vi "ELTA_Ethernet_CMD.vi"(5 "ELTA_Ethernet_Func":T2, 7 "timeout ms":i32=25000, 8 "error in":errorcluster, 11 "CMD in":string) -> (0 "error out":errorcluster, 2 "Response? (00)":bool, 3 "data out":string)   [LabVIEW 2023, in "ELTA.lvlib"]
uses:
  ELTA.lvlib
  DUT_ctrl.ctl
panel:
  in  "TCPIPin":T1={"address"="192.168.100.111", "remote port or service name"=5025, "timeout ms "=10000}
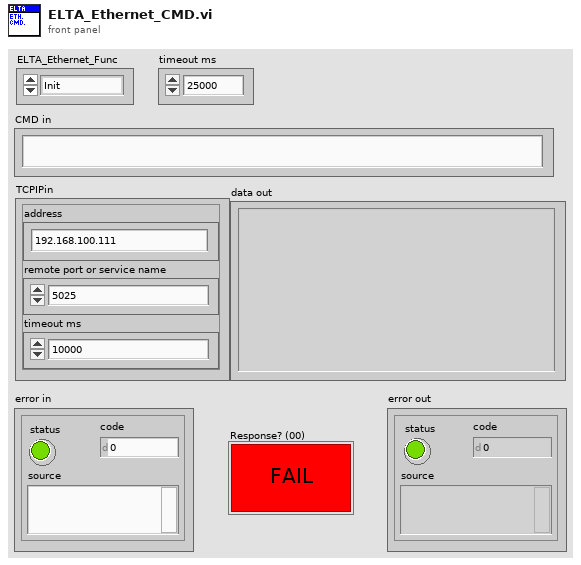
[diagram p1: front panel]
types:
  T1 = cluster{"address":string, "remote port or service name":u16, "timeout ms ":i32}
  T2 = typedef "ELTA.lvlib/DUT_ctrl.ctl" = enum16{"Init", "Close", "CMD"}
  T3 = enum16{"Standard", "Buffered", "CRLF", "Immediate"}
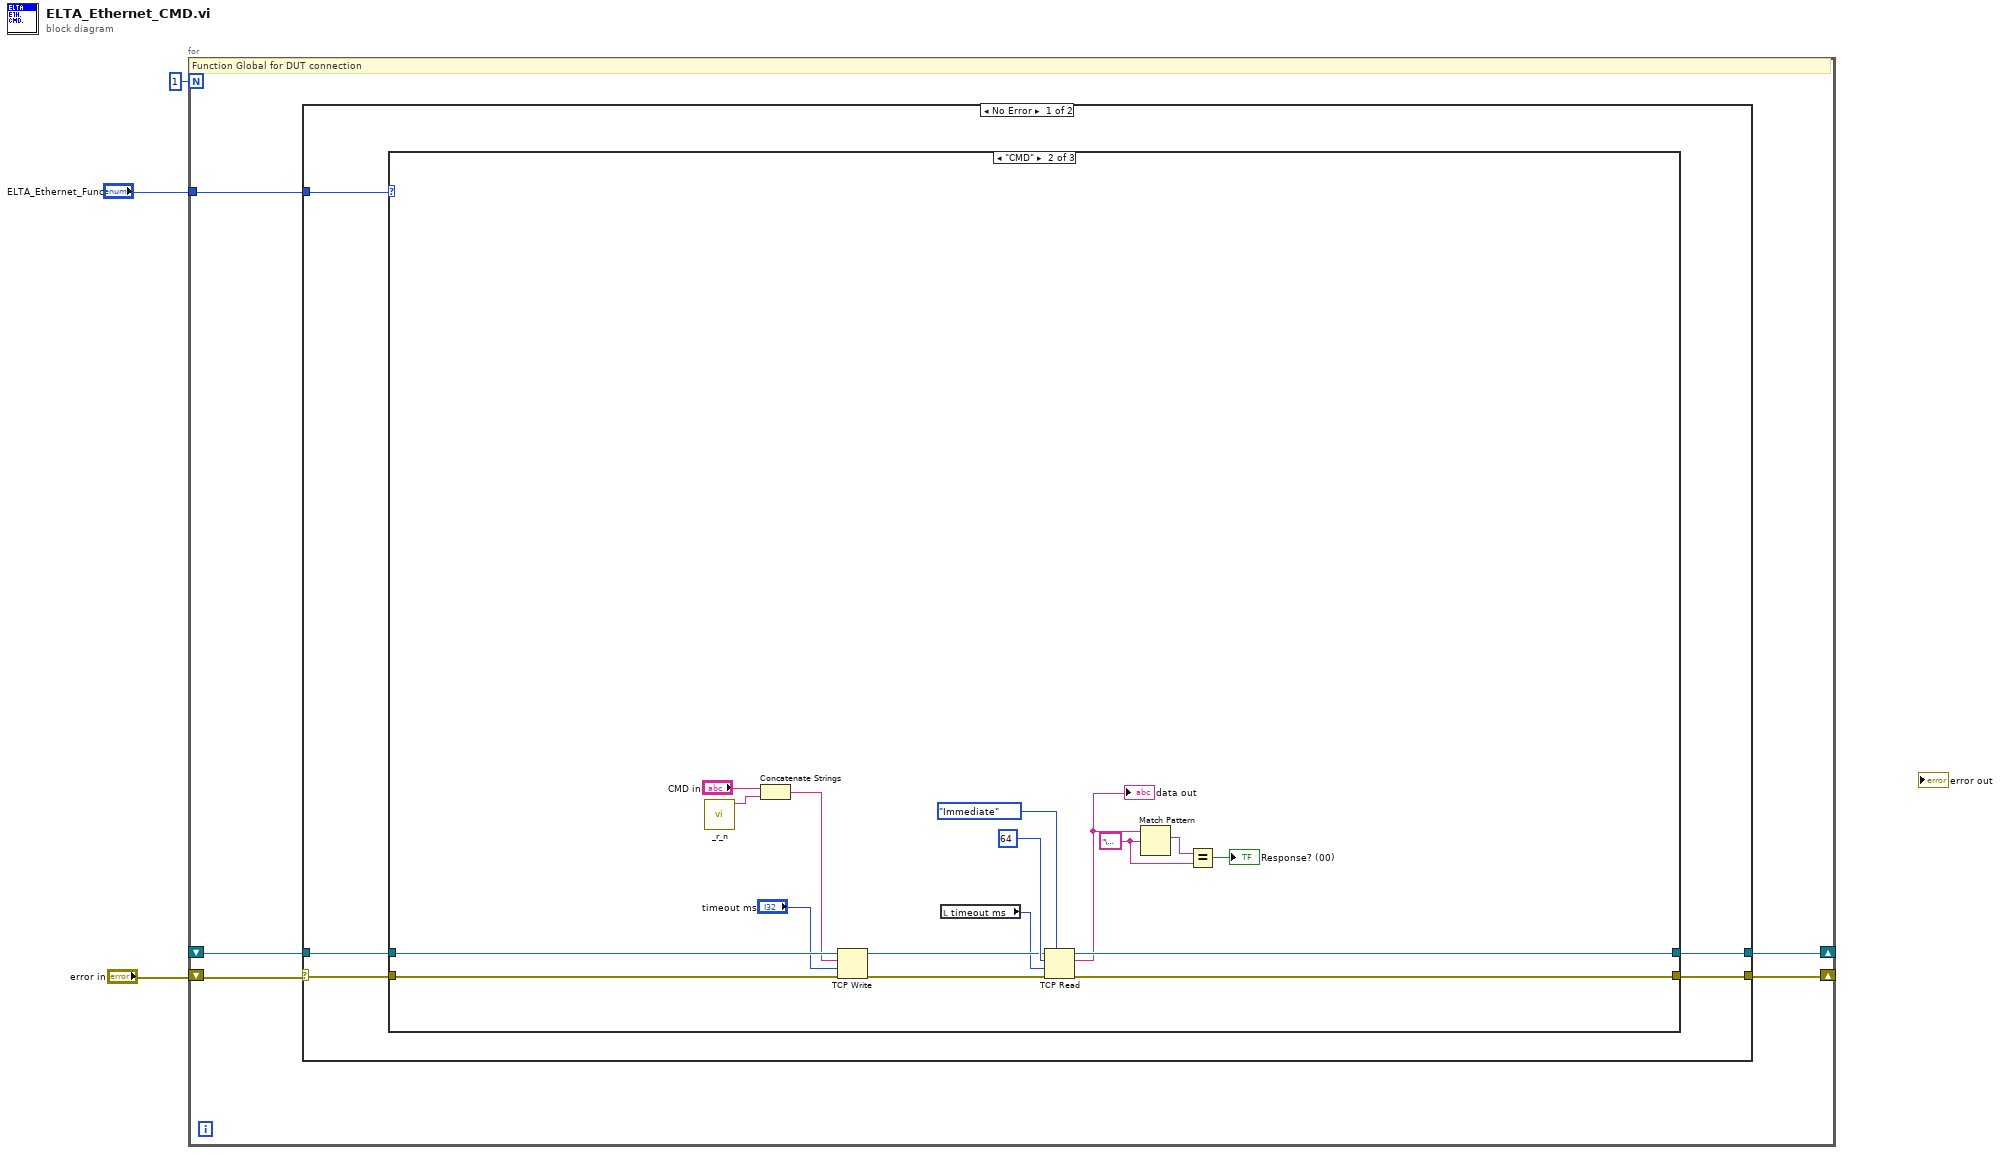
[diagram p0: block diagram]
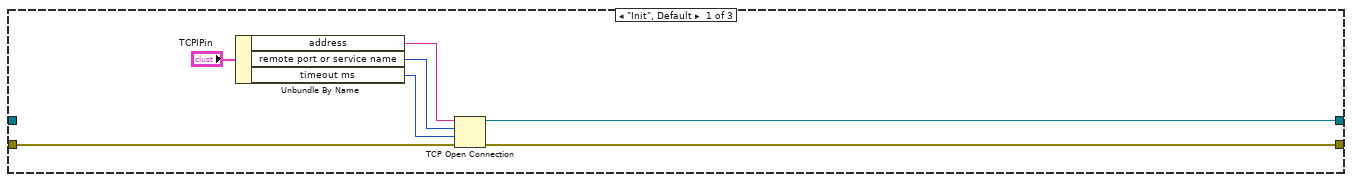
[diagram p2: hidden frame]
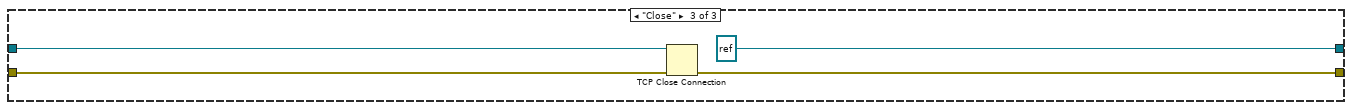
[diagram p3: hidden frame]
diagram:
  n1 = for {
    N: 1 -> [_]
    tunnel: "ELTA_Ethernet_Func" -> [w7]
    shift-right: [w6] -> _
    shift-left: "error in" -> [w8]
    shift-right: [w5] -> _
    shift-left: _ -> [w4]
    # "Function Global for DUT connection"
    n2 = case shown="No Error" w8 {
      selector: w8 -> [w13 w43]
      tunnel: w7 -> [w12 _]
      tunnel: [w11 w43] -> w6
      tunnel: [w10 w42] -> w5
      tunnel: w4 -> [w9 w42]
      frame No Error {
        n3 = case shown="\"CMD\"" w12 {
          tunnel: w13 -> [w19 w37 w40]
          tunnel: [w15 w28 w39] -> w11
          tunnel: [w14 w26 refnum<k5> refnum ("connection ID")] -> w10
          tunnel: w9 -> [_ w36 w38]
          frame "Init", Default {
            n4 = Unbundle By Name("TCPIPin") -> ("address"=w16:string, "remote port or service name"=w17:u16, "timeout ms"=w18:i32)
            n5 = TCP Open Connection(address=w16, remote port or service name=w17, timeout ms (60000)=w18, error in (no error)=w19) -> (connection ID=w14:refnum<k5>, error out=w15:errorcluster)  [unwired: 1 in]
          }
          frame "CMD" {
            w24 = "\u0000" ("string")
            n6 = call "_r_n.vi"() -> ("command"=w33:string)  [unwired: 11 in]
            n7 = Concatenate Strings("CMD in", w33) -> (w34:string)
            n8 = TCP Write(connection ID=w36, data in=w34, error in (no error)=w37, 9:"timeout ms") -> (connection ID out=w27:refnum<k5>, error out=w29:errorcluster)  [unwired: 1 out]
            n9 = local read "timeout ms"() -> (w25:i32)
            n10 = TCP Read(connection ID=w27, bytes to read=64, error in (no error)=w29, 7:T3."Immediate" ("mode (standard)"), 9:w25) -> (connection ID out=w26:refnum<k5>, data out=w22:string, error out=w28:errorcluster)
            "data out" <- w22
            n11 = Match Pattern(string=w22, regular expression=w24) -> (match substring=w23:string)  [unwired: 1 in, 3 out]
            n12 = Equal?(x=w23, y=w24) -> (x = y?=→"Response? (00)":bool)
          }
          frame "Close" {
            n13 = TCP Close Connection(connection ID=w38, error in (no error)=w40) -> (error out=w39:errorcluster)  [unwired: 1 in, 1 out]
          }
        }
      }
      frame Error {
      }
    }
  }
